vi "rotation_to_perm_string.vi"(6 "Angle unit":enum16{"Radians", "Degrees"}(ring)=enum."Degrees", 11 "Rotation matrix (T)":T1 format="%#.3f") -> (3 "Axis permutation and residue":string)   [LabVIEW 2013]
uses:
  <vilib>/Analysis/Matrix/Datatypes/RealMatrix.ctl
  <vilib>/Analysis/Matrix/NI_Matrix.lvlib
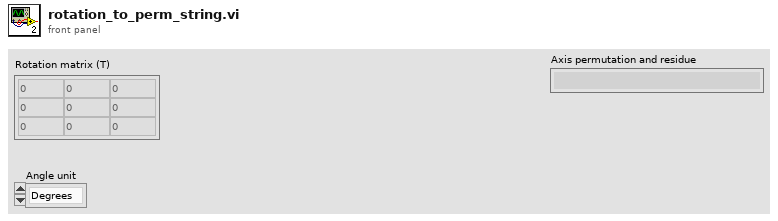
[diagram p1: front panel]
types:
  T1 = typedef "NI_Matrix.lvlib/RealMatrix.ctl" = dbl[][]
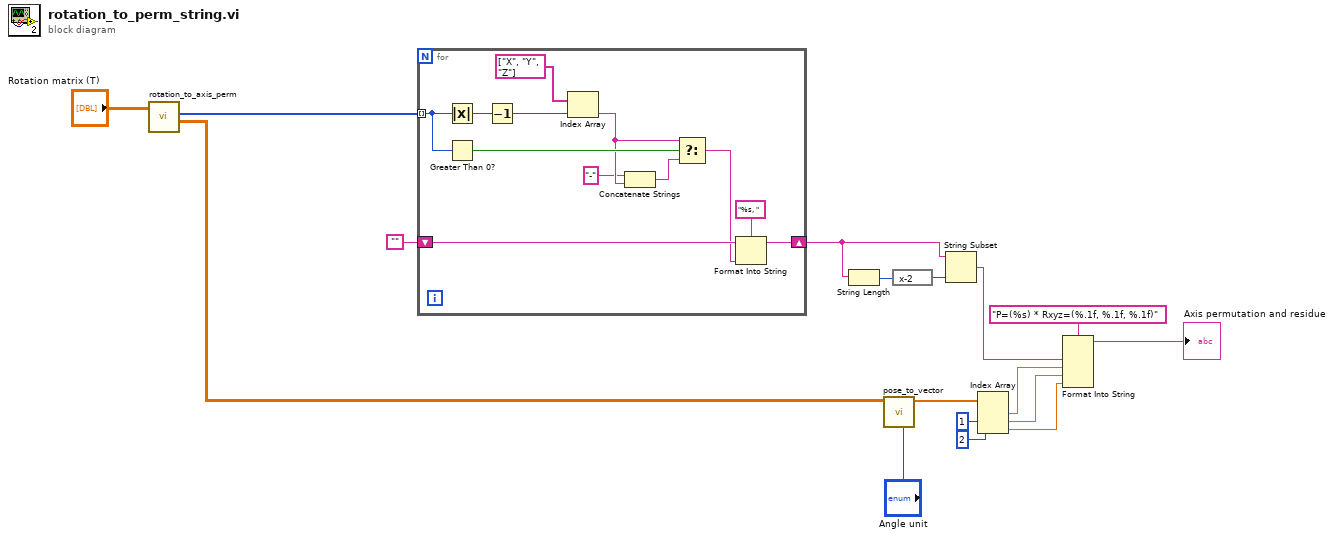
[diagram p0: block diagram]
diagram:
  n1 = call "rotation_to_axis_perm.vi"("Rotation matrix (T)"="Rotation matrix (T)") -> ("Residue matrix (R)"=w16:T1, "Permutation vector"=w15:i32[])  [unwired: 8 in, 1 out]
  n2 = for {
    tunnel: w15 -> [w29] mode=indexing
    shift-right: [w20] -> w11
    shift-left: "" -> [w23]
    n3 = Absolute Value(x=w29) -> (abs(x)=w19:i32)
    n4 = Greater Than 0?(x=w29) -> (x > 0?=w27:bool)
    n5 = Decrement(x=w19) -> (x-1=w18:i32)
    n6 = Index Array(array=string[] ["X", "Y", "Z"], index=w18) -> (element=w26:string)
    n7 = Concatenate Strings("-" ("string"), w26) -> (w25:string)
    n8 = Select(t=w26, s=w27, f=w25) -> (s? t:f=w21:string)
    n9 = Format Into String(format string="%s, ", initial string=w23, w21) -> (resulting string=w20:string)  [unwired: 1 in, 1 out]
  }
  n10 = String Length(string=w11) -> (length=w13:i32)
  n11 = call "pose_to_vector.vi"("Angle unit"="Angle unit", "Pose"=w16) -> ("Pose vector"=w6:dbl[])  [unwired: 9 in]
  n12 = expression code="x-2"(w13) -> (w12:i32)
  n13 = String Subset(string=w11, length (rest)=w12) -> (substring=w9:string)  [unwired: 1 in]
  n14 = Index Array(array=w6, index #2=1 ("index"), index #3=2 ("index")) -> (element #1=w5:dbl, element #2=w3:dbl, element #3=w4:dbl)  [unwired: 1 in]
  n15 = Format Into String(format string="P=(%s) * Rxyz=(%.1f, %.1f, %.1f)", w9, w5, w3, w4) -> (resulting string=→"Axis permutation and residue":string)  [unwired: 2 in, 1 out]
